vi "SelectMenu5.vi"(0 "XRef":T18, 1 "Tag":T13, 2 "Point":T16, 3 "Menu Type":T15, 4 "State In":T1) -> (14 "Reply":T12, 15 "Handled?":T14, 16 "Multi Object Popup Options":T11, 17 "Fatal Error Out":T10, 18 "State Out":T1)   [LabVIEW 2020, in "FlexBlock.xnode"]
uses:
  FlexBlock.xnode
  <vilib>/XNodeSupport/XNodeXNodeRef.ctl
  <vilib>/XNodeSupport/XNodeString.ctl
  <vilib>/XNodeSupport/XNodePoint.ctl
  <vilib>/XNodeSupport/XNodeInt.ctl
  <vilib>/XNodeSupport/XNodeMenuType.ctl
  State.ctl
  FlexBlocks/Type Descriptor.ctl
  FlexBlocks/Terminal Direction.ctl
  FlexBlocks/Value Mode.ctl
  FlexBlocks/Terminal State.ctl
  FlexBlocks/Special Terminal.ctl
  FlexBlocks/Errors.ctl
  <vilib>/picture/picture.llb/imagedata.ctl
  FlexBlocks/Calculated Sizes.ctl
  <vilib>/XNodeSupport/XNodeStringArray.ctl
  <vilib>/XNodeSupport/XNodeBool.ctl
  <vilib>/XNodeSupport/XNodeMultiObjectPopupOptions.ctl
  <vilib>/XNodeSupport/XNodeErrorCluster.ctl
  <vilib>/XNodeSupport/NI_XNodeSupport.lvlib
  FlexBlocks/Menu Action.ctl
  FlexBlocks/FlexBlocks.lvlib
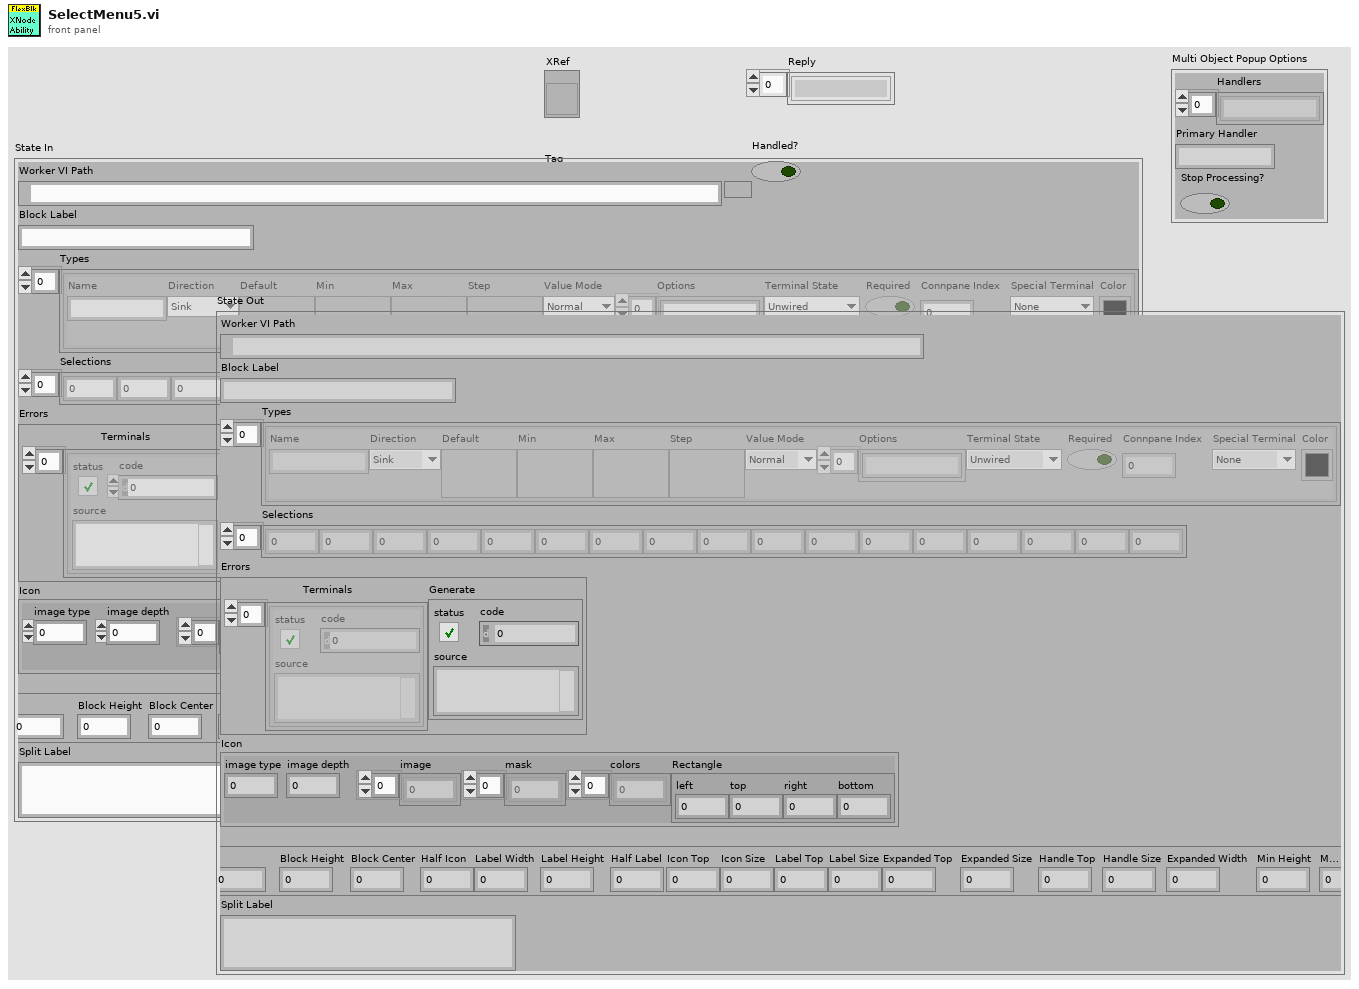
[diagram p1: front panel]
types:
  T1 = typedef "FlexBlock.xnode/State.ctl" = cluster{"Worker VI Path":path, "Block Label":string, "Types":T2[], "Selections":i32[], "Errors":T7, "Icon":T8, "Calcd Sizes":T9, "Split Label":string}
  T2 = typedef "FlexBlocks.lvlib/Type Descriptor.ctl" = cluster{"Name":string, "Direction":T3, "Default":variant, "Min":variant, "Max":variant, "Step":variant, "Value Mode":T4, "Options":string[], "Terminal State":T5, "Required":bool, "Connpane Index":i32, "Special Terminal":T6, "Color":u32}
  T3 = typedef "FlexBlocks.lvlib/Terminal Direction.ctl" = enum16{"Sink", "Source"}
  T4 = typedef "FlexBlocks.lvlib/Value Mode.ctl" = enum16{"Normal", "Range", "Select"}
  T5 = typedef "FlexBlocks.lvlib/Terminal State.ctl" = enum16{"Unwired", "BadType", "BadRef", "Channel", "Value", "Control Ref"}
  T6 = typedef "FlexBlocks.lvlib/Special Terminal.ctl" = enum16{"None", "Action", "Init", "Tag", "State in", "State out", "Error"}
  T7 = typedef "FlexBlocks.lvlib/Errors.ctl" = cluster{"Terminals":errorcluster[], "Generate":errorcluster}
  T8 = typedef "imagedata.ctl" = cluster{"image type":i32, "image depth":i32, "image":u8[], "mask":u8[], "colors":u32[], "Rectangle":cluster{"left":i16, "top":i16, "right":i16, "bottom":i16}}
  T9 = typedef "FlexBlocks.lvlib/Calculated Sizes.ctl" = cluster{"Text Width":i32, "Text Height":i32, "Half Text":i32, "Block Width":i32, "Block Height":i32, "Block Center":i32, "Half Icon":i32, "Label Width":i32, "Label Height":i32, "Half Label":i32, "Icon Top":i32, "Icon Size":i32, "Label Top":i32, "Label Size":i32, "Expanded Top":i32, "Expanded Size":i32, "Handle Top":i32, "Handle Size":i32, "Expanded Width":i32, "Min Height":i32, "Max Height":i32}
  T10 = typedef "NI_XNodeSupport.lvlib/XNodeErrorCluster.ctl" = errorcluster
  T11 = typedef "NI_XNodeSupport.lvlib/XNodeMultiObjectPopupOptions.ctl" = cluster{"Handlers":T12, "Primary Handler":T13, "Stop Processing?":T14}
  T12 = typedef "NI_XNodeSupport.lvlib/XNodeStringArray.ctl" = T13[]
  T13 = typedef "NI_XNodeSupport.lvlib/XNodeString.ctl" = string
  T14 = typedef "NI_XNodeSupport.lvlib/XNodeBool.ctl" = bool
  T15 = typedef "NI_XNodeSupport.lvlib/XNodeMenuType.ctl" = enum32{"Single Object Operate", "Single Object Popup", "Multi Object Popup Master", "Multi Object Popup Other"}
  T16 = typedef "NI_XNodeSupport.lvlib/XNodePoint.ctl" = cluster{"H":T17, "V":T17}
  T17 = typedef "NI_XNodeSupport.lvlib/XNodeInt.ctl" = i32
  T18 = typedef "NI_XNodeSupport.lvlib/XNodeXNodeRef.ctl" = refnum<vi>
  T19 = typedef "FlexBlocks.lvlib/Menu Action.ctl" = enum16{"ITEM_SEL", "VAL_SEL"}
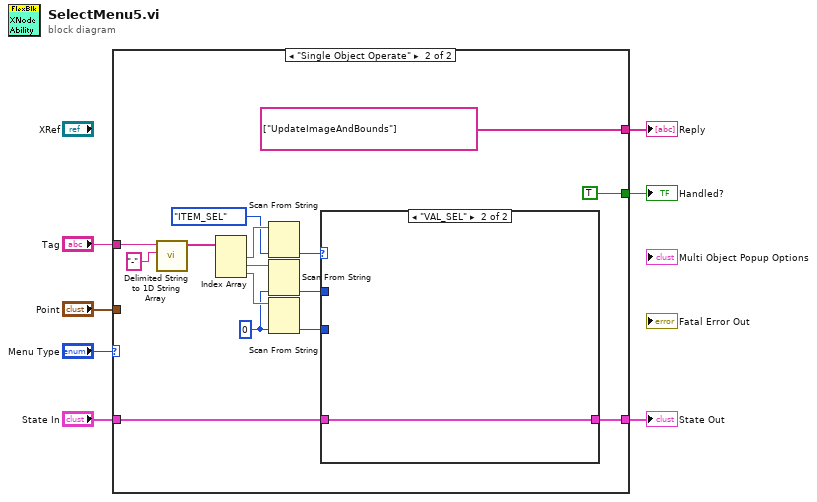
[diagram p0: block diagram]
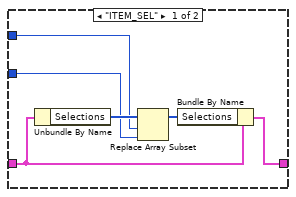
[diagram p3: hidden frame]
diagram:
  n1 = case shown="\"Single Object Operate\"" "Menu Type" {
    tunnel: "State In" -> [w8 w13]
    tunnel: "Point" -> [_ _]
    tunnel: "Tag" -> [_ w21]
    tunnel: [_ T12 ["UpdateImageAndBounds"] ("Reply")] -> w3
    tunnel: [_ TRUE] -> w2
    tunnel: [w8 w9] -> w1
    frame Default {
    }
    frame "Single Object Operate" {
      w14 = 0 ("default value 1")
      n2 = call <vilib>:"Delimited String to 1D String Array.vi"("delimiter"="-", "delimited string"=w21) -> ("string array"=w19:string[])  [unwired: 9 in]
      n3 = Index Array(array=w19) -> (element #1=w18:string, element #2=w16:string, element #3=w15:string)  [unwired: 3 in]
      n4 = Scan From String(input string=w18, default 1=Menu_Action."ITEM_SEL" ("Menu Action")) -> (output 1=w12:T19)  [unwired: 3 in, 3 out]
      n5 = Scan From String(input string=w16, default 1=w14) -> (output 1=w11:i32)  [unwired: 3 in, 3 out]
      n6 = Scan From String(input string=w15, default 1=w14) -> (output 1=w10:i32)  [unwired: 3 in, 3 out]
      n7 = case shown="\"VAL_SEL\"" w12 {
        tunnel: w13 -> [w26 w30]
        tunnel: w11 -> [w28 _]
        tunnel: w10 -> [w27 _]
        tunnel: [w24 w30] -> w9
        frame "ITEM_SEL" {
          n8 = Unbundle By Name(w26) -> ("Selections"=w29:i32[])
          n9 = Replace Array Subset(array=w29, new element=w27, index=w28) -> (w25:i32[])
          n10 = Bundle By Name(cluster=w26, "Selections"=w25) -> (w24:T1)
        }
        frame "VAL_SEL" {
        }
      }
    }
  }
  "Reply" <- w3
  "Handled?" <- w2
  "State Out" <- w1
